vi "FCI_Cam_0_Coordinate_System.vi"(0 "Image Out":T7(plugin-control), 1 "ROI Descriptor":T1 {"Contours"."Type" items=["No Selection", "Point", "Line", "Rectangle", "Oval", "Polygon", "Freehand Region", "Annulus", "Unused2", "Unused3", "Broken Line", "Freehand Line", "Rotated Rectangle"]}, 5 "Edge Options":T3={"Edge Polarity"=2, "Kernel Size"=3, "Width"=3, "Minimum Edge Strength"=50.0, "Interpolation Type"=enum."Zero Order", "Data Processing Method"=enum."Average"} {"Edge Polarity" items=["All Edges", "Rising Edges", "Falling Edges"]; "Minimum Edge Strength" format="%.2f"; "Width" step=2; "Kernel Size" step=2}, 7 "Line Options":T5={"Number of Lines"=1, "Type"=enum."First Edge Rake", "Min. Score"=10.0, "Max. Score"=1000.0, "Orientation"=0.0, "Angle Range"=70.0, "Angle Tolerance"=10.0, "Step Size"=12, "Min. SNR (db)"=0.0, "Min. Points (%)"=25.0, "Hough Iterations"=5} {"Min. Points (%)" min=0.0 max=100.0; "Min. SNR (db)" min=0.0; "Max. Score" min=0.0 max=1024.0; "Min. Score" min=0.0 max=1024.0 step=1.0}, 9 "Search Direction":u32(ring) items=["Left to Right", "Right to Left", "Top to Bottom", "Bottom to Top"], 11 "error in (no error)":errorcluster, 12 "ParallelLines":cluster{"First":i32, "Second":i32, "Third":i32}) -> (4 "Coordinate System":T2 {"Axis Reference" items=["Direct", "Indirect"]; "Angle (deg)" format="%.2f"; "Origin"."Y" format="%.2f"; "Origin"."X" format="%.2f"}, 15 "error out":errorcluster)   [LabVIEW 2015]
uses:
  <vilib>/vision/Measure.llb/Straight Edge Options.ctl
  <vilib>/vision/Measure.llb/Straight Edge Process.ctl
  <vilib>/vision/Measure.llb/Edge Options.ctl
  <vilib>/vision/Measure.llb/Edge Polarity.ctl
  <vilib>/vision/NI_Vision_Development_Module.lvlib
  FrameworkOverrides/Algorithm.lvclass
panel:
  out "Edge Coordinates":cluster{"X":sgl, "Y":sgl}[](array[cluster]) {"Y" format="%.2f"; "X" format="%.2f"}
  in  "Settings":T8={"Contrast"=40, "Filter width"=4, "Steepness"=2, "Subsampling Ratio"=5, "Show Search Area"=FALSE, "Show Search Lines"=FALSE, "Show Edges Found"=FALSE, "Show Result"=TRUE}
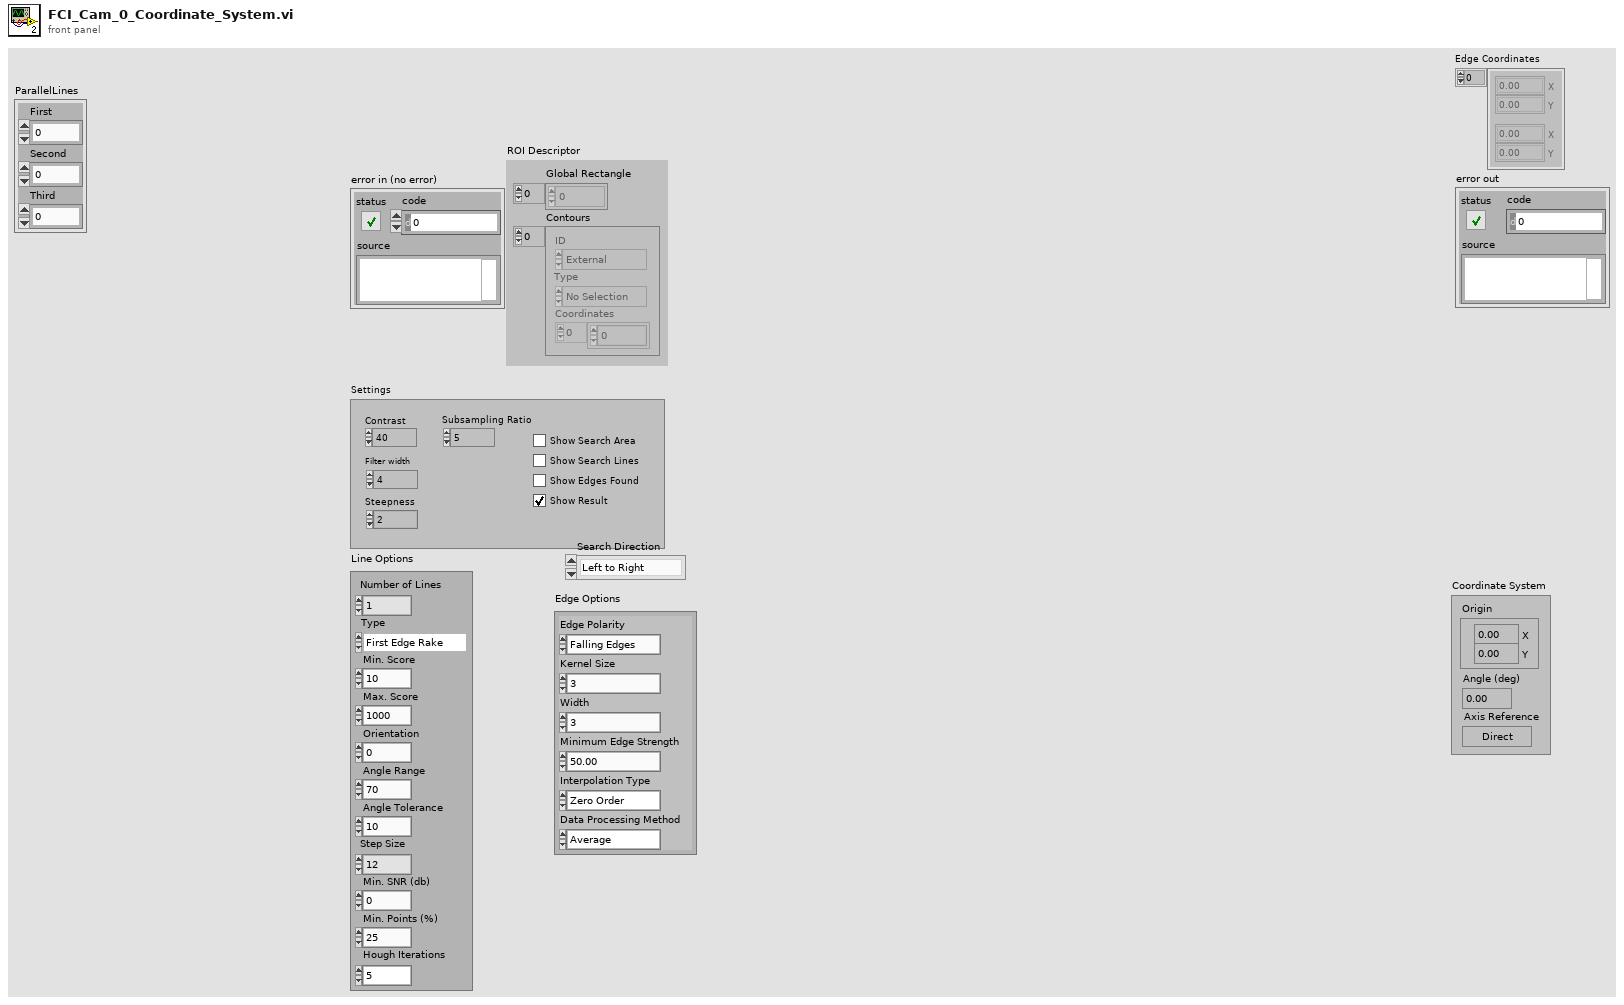
[diagram p1: front panel]
types:
  T1 = typedef "ROI Descriptor" = cluster{"Global Rectangle":i32[], "Contours":cluster{"ID":enum32{"External", "Internal"}, "Type":u32, "Coordinates":i32[]}[]}
  T2 = cluster{"Origin":cluster{"X":sgl, "Y":sgl}, "Angle (deg)":sgl, "Axis Reference":u32}
  T3 = typedef "Edge Options.ctl" = cluster{"Edge Polarity":T4, "Kernel Size":u32, "Width":u32, "Minimum Edge Strength":sgl, "Interpolation Type":enum32{"Zero Order", "Bilinear", "Quadratic", "Cubic", "Bilinear Fixed"}, "Data Processing Method":enum32{"Average", "Median"}}
  T4 = typedef "Edge Polarity.ctl" = u32
  T5 = typedef "Straight Edge Options.ctl" = cluster{"Number of Lines":i32, "Type":T6, "Min. Score":dbl, "Max. Score":dbl, "Orientation":dbl, "Angle Range":dbl, "Angle Tolerance":dbl, "Step Size":u32, "Min. SNR (db)":dbl, "Min. Points (%)":dbl, "Hough Iterations":i32}
  T6 = typedef "Straight Edge Process.ctl" = enum32{"First Edge Rake", "Best Edge Rake", "Hough Edge Rake", "First Edge Projection", "Best Edge Projection"}
  T7 = typedef "IMAQ Image.ctl" = refnum<image>
  T8 = cluster{"Contrast":i32, "Filter width":i32, "Steepness":i32, "Subsampling Ratio":u32, "Show Search Area":bool, "Show Search Lines":bool, "Show Edges Found":bool, "Show Result":bool}
  T9 = typedef "IMAQ Rectangle" = cluster{"Left":i32, "Top":i32, "Right":i32, "Bottom":i32, "Rotation":dbl}
  T10 = cluster{"Point1 (Pixels)":cluster{"X":sgl, "Y":sgl}, "Point2 (Pixels)":cluster{"X":sgl, "Y":sgl}, "Point1 (Real-World)":cluster{"X":sgl, "Y":sgl}, "Point2 (Real-World)":cluster{"X":sgl, "Y":sgl}, "Angle (Pixel)":dbl, "Angle (Real-World)":dbl, "Score":dbl, "Straightness":dbl, "Average SNR (db)":dbl, "Calibration Valid":bool}[]
  T11 = cluster{"Point1 (Pixels)":cluster{"X":sgl, "Y":sgl}, "Point2 (Pixels)":cluster{"X":sgl, "Y":sgl}, "Point1 (Real-World)":cluster{"X":sgl, "Y":sgl}, "Point2 (Real-World)":cluster{"X":sgl, "Y":sgl}, "Angle (Pixel)":dbl, "Angle (Real-World)":dbl, "Score":dbl, "Straightness":dbl, "Average SNR (db)":dbl, "Calibration Valid":bool}
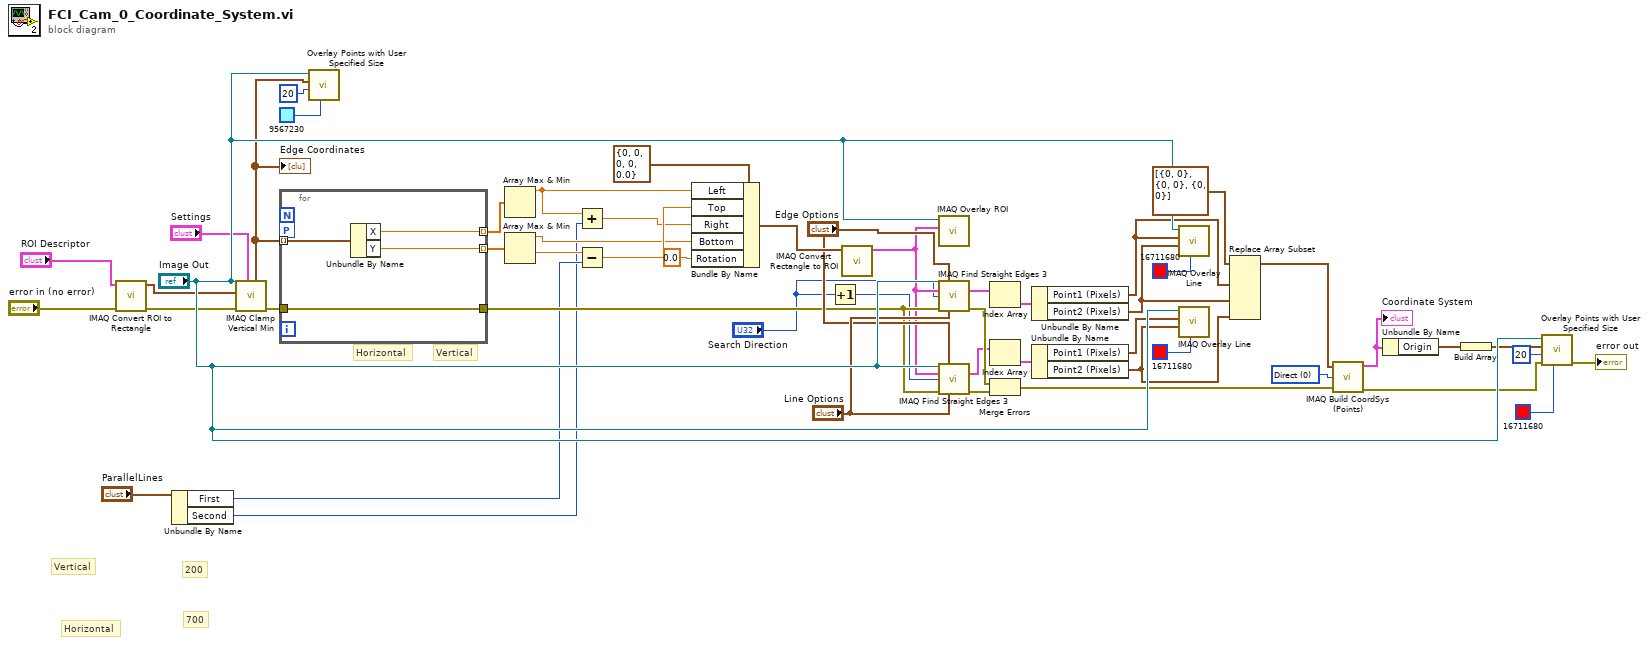
[diagram p0: block diagram]
diagram:
  w19 = u32 0 items=["Direct", "Indirect"] ("Axis Reference")
  # "Horizontal"
  # "Vertical"
  # "700"
  # "200"
  # "Horizontal"
  # "Vertical"
  n1 = call "IMAQ Convert ROI to Rectangle"("error in (no error)"="error in (no error)", "ROI Descriptor"="ROI Descriptor") -> ("error out"=w11:errorcluster, "Rectangle"=w51:T9)  [unwired: 7 in]
  n2 = Unbundle By Name("ParallelLines") -> ("First"=w4:i32, "Second"=w3:i32)
  n3 = call "IMAQ Clamp Vertical Min"("Settings"="Settings", "error in (no error)"=w11, "Rectangle"=w51, "Image"="Image Out") -> ("error out"=w45:errorcluster, "Edge Coordinates"=w48:cluster{"X":sgl, "Y":sgl}[])  [unwired: 3 in, 3 out]
  "Edge Coordinates" <- w48
  n4 = for {
    tunnel: w48 -> [w56] mode=indexing
    tunnel: [w55] -> w47 mode=indexing
    tunnel: [w54] -> w46 mode=indexing
    tunnel: w45 -> [w53]
    tunnel: [w53] -> w32
    workers-P: _ -> [_]
    n5 = Unbundle By Name(w56) -> ("X"=w55:sgl, "Y"=w54:sgl)
  }
  n6 = call "Overlay Points with User Specified Size.vi"("Color"=u32 9567230, "Point Diameter (5)"=u32 20, "Points"=w48, "Image In"="Image Out") -> ()  [unwired: 6 in, 2 out]
  n7 = Array Max & Min(array=w47) -> (max value=w37:sgl)  [unwired: 3 out]
  n8 = Array Max & Min(array=w46) -> (max value=w40:sgl, min value=w44:sgl)  [unwired: 2 out]
  n9 = Add(x=w37, y=w3) -> (x+y=w38:sgl)
  n10 = Subtract(x=w44, y=w4) -> (x-y=w41:sgl)
  n11 = Bundle By Name(cluster=T9 {"Left"=0, "Top"=0, "Right"=0, "Bottom"=0, "Rotation"=0.0} ("Rectangle"), "Left"=w37, "Top"=w41, "Right"=w38, "Bottom"=w40, "Rotation"=0.0) -> (w39:T9)
  n12 = Increment(x="Search Direction") -> (x+1=w7:u32)
  n13 = call "IMAQ Convert Rectangle to ROI"("Rectangle"=w39) -> ("ROI Descriptor"=w25:T1)  [unwired: 8 in, 1 out]
  n14 = call "IMAQ Overlay ROI"("ROI Descriptor"=w25, "Image"="Image Out") -> ()  [unwired: 8 in, 2 out]
  n15 = call "IMAQ Find Straight Edges 3"("Image"="Image Out", "Edge Options"="Edge Options", "ROI Descriptor"=w25, "Search Direction"="Search Direction", "error in (no error)"=w32, "Line Options"="Line Options") -> ("Straight Edges"=w31:T10, "error out"=w34:errorcluster)  [unwired: 5 in, 3 out]
  n16 = call "IMAQ Find Straight Edges 3"("Image"="Image Out", "Edge Options"="Edge Options", "ROI Descriptor"=w25, "Search Direction"=w7, "error in (no error)"=w32, "Line Options"="Line Options") -> ("Straight Edges"=w28:T10, "error out"=w33:errorcluster)  [unwired: 5 in, 3 out]
  n17 = Index Array(array=w31) -> (element=w30:T11)  [unwired: 1 in]
  n18 = Index Array(array=w28) -> (element=w29:T11)  [unwired: 1 in]
  n19 = Merge Errors(w34, w33) -> (w13:errorcluster)
  n20 = Unbundle By Name(w30) -> ("Point1 (Pixels)"=w23:cluster{"X":sgl, "Y":sgl}, "Point2 (Pixels)"=w22:cluster{"X":sgl, "Y":sgl})
  n21 = Unbundle By Name(w29) -> ("Point1 (Pixels)"=w21:cluster{"X":sgl, "Y":sgl}, "Point2 (Pixels)"=w12:cluster{"X":sgl, "Y":sgl})
  n22 = call "IMAQ Overlay Line"("Color"=u32 16711680, "End Point"=w22, "Start Point"=w23, "Image"="Image Out") -> ()  [unwired: 6 in, 2 out]
  n23 = call "IMAQ Overlay Line"("Color"=u32 16711680, "End Point"=w12, "Start Point"=w21, "Image"="Image Out") -> ()  [unwired: 6 in, 2 out]
  n24 = Replace Array Subset(array=cluster{"X":i32, "Y":i32}[] [{"X"=0, "Y"=0}, {"X"=0, "Y"=0}, {"X"=0, "Y"=0}] ("Reference Points"), new element #1=w23, new element #2=w22, new element #3=w12) -> (w20:cluster{"X":i32, "Y":i32}[])  [unwired: 3 in]
  n25 = call "IMAQ Build CoordSys (Points)"("Reference Points"=w20, "Axis Reference"=w19, "error in (no error)"=w13) -> ("Coordinate System"=w18:T2, "error out"=w2:errorcluster)  [unwired: 2 in]
  "Coordinate System" <- w18
  n26 = Unbundle By Name(w18) -> ("Origin"=w17:cluster{"X":sgl, "Y":sgl})
  n27 = Build Array(w17) -> (w16:cluster{"X":sgl, "Y":sgl}[])
  n28 = call "Overlay Points with User Specified Size.vi"("Color"=u32 16711680, "error in"=w2, "Point Diameter (5)"=u32 20, "Points"=w16, "Image In"="Image Out") -> ("error out"=→"error out":errorcluster)  [unwired: 5 in, 1 out]
